vi "Performance Test.vi"() -> ()   [LabVIEW 2021]
uses:
  ChannelCommon/typedef/Benchmark Stats.ctl
  CIFChannels/Typedef/Direction.ctl
  CIF_NIChn_Fifo_U8.lvclass
  D:/dev/Packages/Channel_Manager/src/CIFChannels/CIFChannels.lvclass
  ChannelCommon/typedef/FIFO Config.ctl
  <vilib>/Platform/TimedLoop/XDataNode/timing_clust.ctl
  <vilib>/Platform/TimedLoop/XDataNode/nitl_modes.ctl
  <vilib>/Platform/TimedLoop/XDataNode/wakeup.ctl
  ChannelCommon/typedef/TimeStamps.ctl
  CIFChannels/CIFChannels.lvclass/CIFChannels.ctl
  <vilib>/CIF Foundation/CIF Utilities/Statistics/I64/Stats_I64_CIF_U.lvclass/Stats_I64_CIF_U.ctl
  <vilib>/CIF Foundation/CIF Utilities/DataTypes/Flatten U64.vi
  <vilib>/CIF Foundation/CIF Utilities/Statistics/I64/Get Stats.vi
  <vilib>/Platform/TimedLoop/XDataNode/XDataNode.xnode
  <vilib>/Platform/TimedLoop/XDataNode/XDNodeRunTimeDep.lvlib
  CIFChannels/CIFChannels.lvclass
  ChannelCommon/ChannelCommon.lvlib
panel:
  out "Flatten (us) TO":T1
  out "Channel R/W (us) TO":T1
  out "Flatten (us)":T1
  out "Channel R/W (us)":T1
  out "avg TO":dbl
  out "max TO":dbl
  out "timed out? 3":bool
  out "timed out?":bool
  out "avg channel":dbl
  out "max channel":dbl
  out "pass":bool
  out "error out":errorcluster
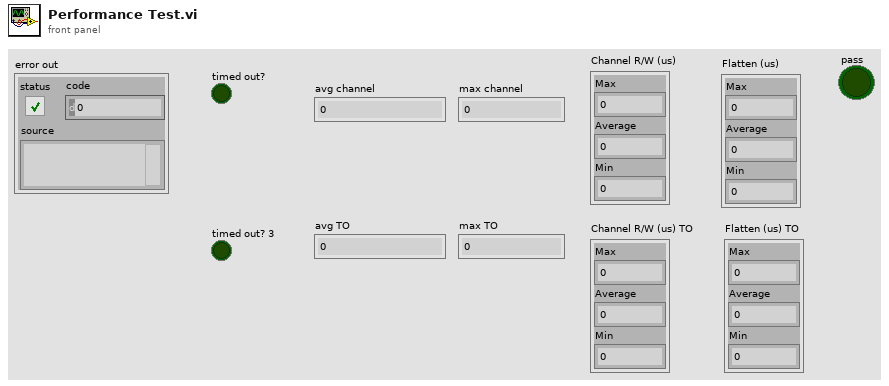
[diagram p1: front panel]
types:
  T1 = typedef "ChannelCommon.lvlib/Benchmark Stats.ctl" = cluster{"Max":i64, "Average":dbl, "Min":i64}
  T2 = typedef "ChannelCommon.lvlib/FIFO Config.ctl" = cluster{"Max Bytes/Msg":u64, "Max Msg/FIFO":u64, "Flags":u64}
  T3 = typedef "CIFChannels.lvclass/Direction.ctl" = enum16{"Publisher", "Subscriber"}
  T4 = typedef "ChannelCommon.lvlib/TimeStamps.ctl" = cluster{"ClockID":u8, "T0":i64, "T_Out":i64}
  T5 = typedef "XDNodeRunTimeDep.lvlib/timing_clust.ctl" = cluster{"Expected End [f-1]":u64, "Actual End [f-1]":u64, "Finished Late? [f-1]":bool, "Expected End [i-1]":u64, "Actual End [i-1]":u64, "Finished Late? [i-1]":bool, "Expected Start [i]":u64, "Actual Start [i]":u64, "Expected Start [f]":u64, "Actual Start [f]":u64, "Source Name":string, "Structure Name":string, "Period":i64, "Deadline":i64, "Offset":i64, "Start":i64, "Priority":i32, "Timeout":i32, "Mode":T6, "Wakeup Reason":T7, "Error":errorcluster, "Source Type":string, "Secondary Source Type":string, "Global End Time":u64, "Global Start Time":u64, "Frame Duration":u64, "Iteration Duration":u64, "Assigned CPU":i32, "I/O Scan Engine Mode":u32}
  T6 = typedef "XDNodeRunTimeDep.lvlib/nitl_modes.ctl" = enum32{"No Change", "Process missed periods, maintain original phase", "Discard missed periods, maintain original phase", "Process missed periods, ignore original phase", "Discard missed periods, ignore original phase"}
  T7 = typedef "XDNodeRunTimeDep.lvlib/wakeup.ctl" = enum32{"Normal", "Aborted", "Asynchronous wakeup", "Timing source error", "Timed loop error", "Timeout"}
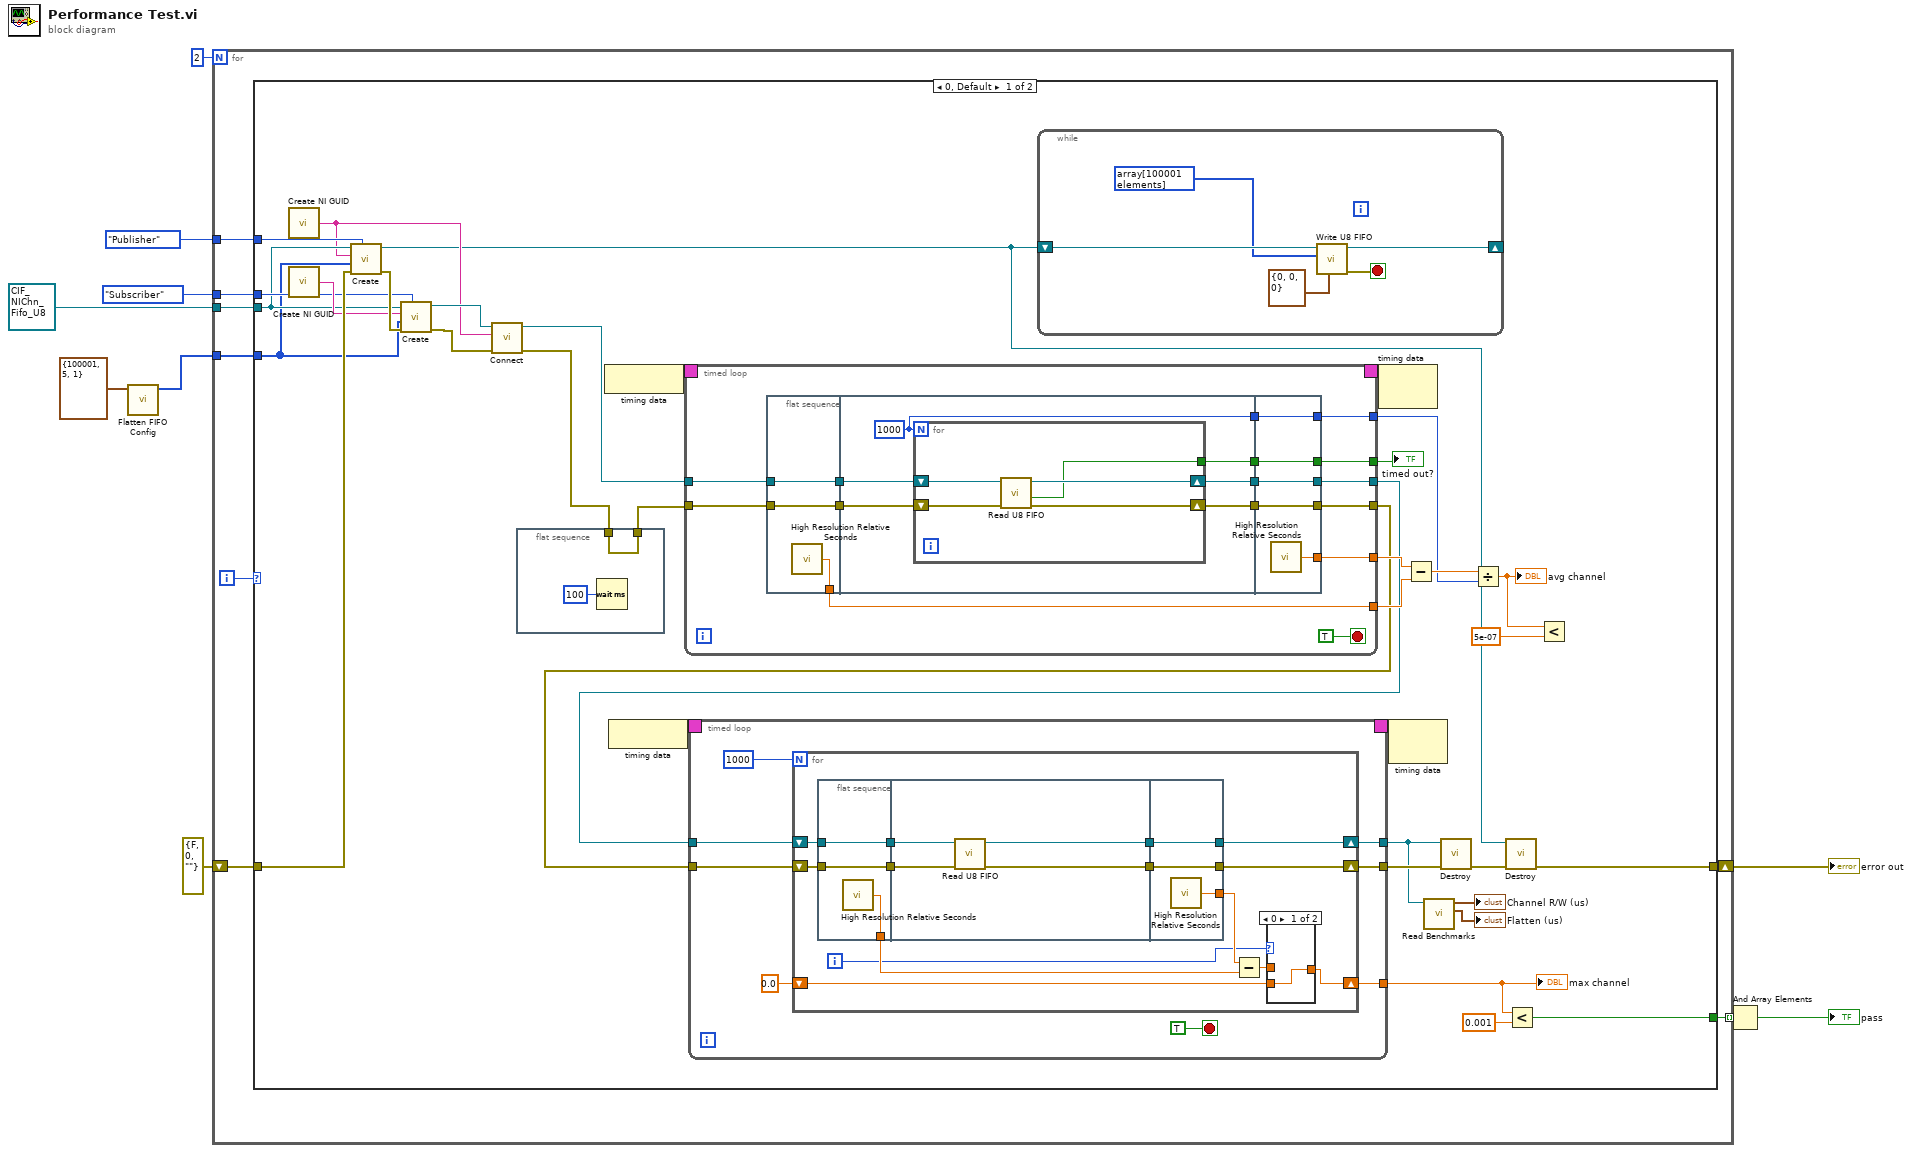
[diagram p0: block diagram]
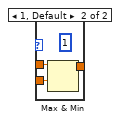
[diagram p2: hidden frame]
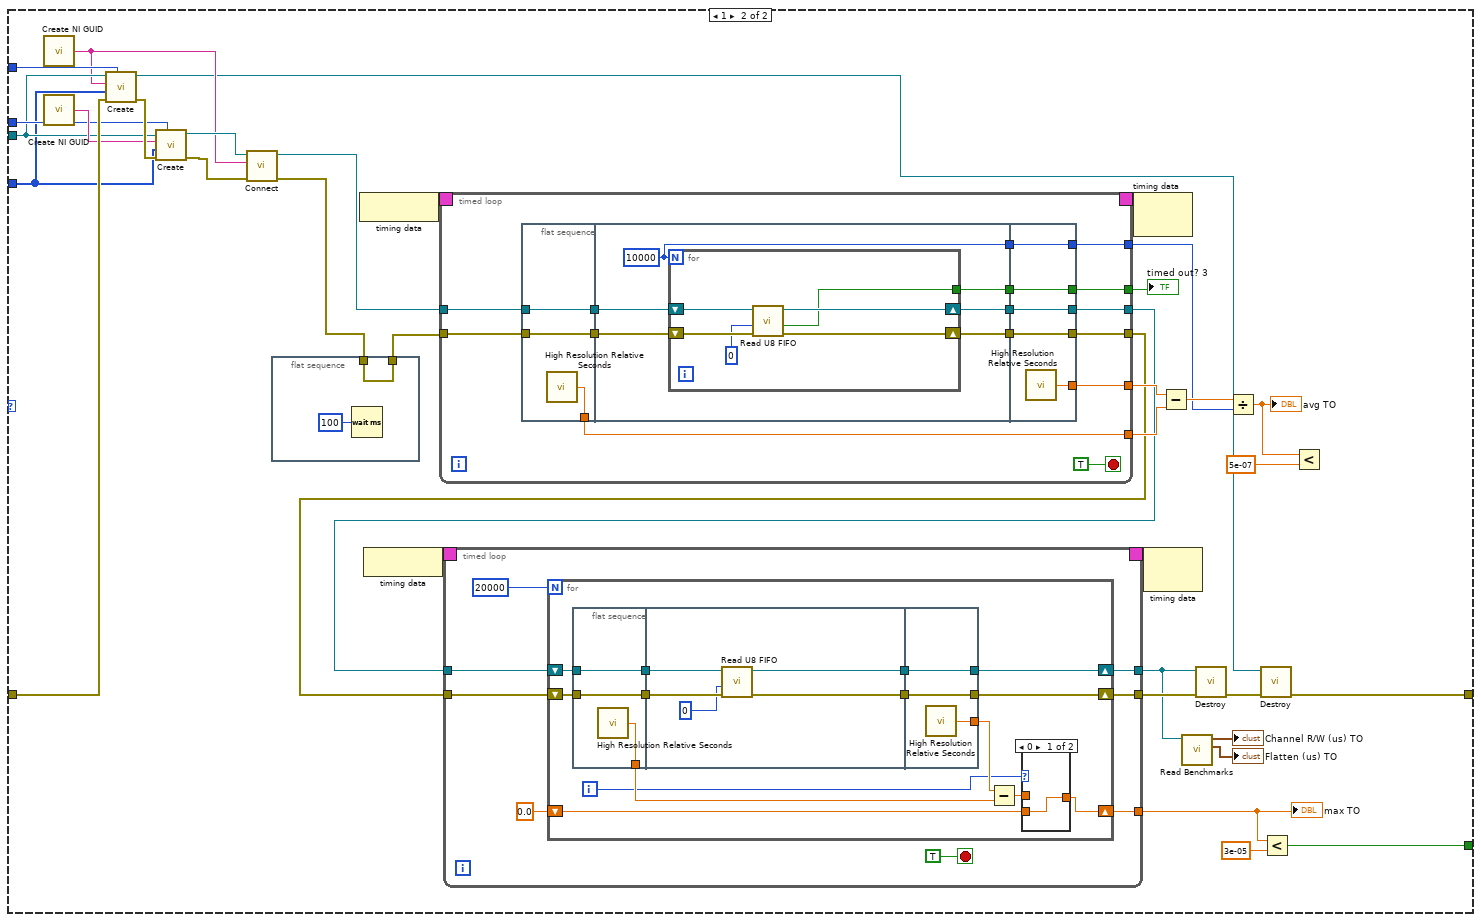
[diagram p3: hidden frame]
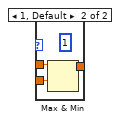
[diagram p4: hidden frame]
diagram:
  n1 = call "Flatten FIFO Config.vi"("FIFO Config in"=T2 {"Max Bytes/Msg"=100001, "Max Msg/FIFO"=5, "Flags"=1}) -> ("Flattened FIFO Config"=w1:u8[])  [unwired: 10 in]
  n2 = for {
    N: 2 -> [_]
    tunnel: [w18] -> w8 mode=indexing
    shift-right: [w17] -> w10
    shift-left: errorcluster {"status"=FALSE, "code"=0, "source"=""} ("error out") -> [w15]
    tunnel: Direction."Publisher" ("Direction") -> [w14]
    tunnel: Direction."Subscriber" ("Direction") -> [w13]
    tunnel: refnum<class "CIF_NIChn_Fifo_U8.lvclass"> refnum ("CIF_NIChn_Fifo_Power.lvclass") -> [w12]
    tunnel: w1 -> [w11]
    i -> [w16]
    n3 = case shown="0, Default" w16 {
      tunnel: [w40 w161] -> w18
      tunnel: [w25 w146] -> w17
      tunnel: w15 -> [w38 w159]
      tunnel: w14 -> [w36 w157]
      tunnel: w13 -> [w35 w156]
      tunnel: w12 -> [w34 w155]
      tunnel: w11 -> [w30 w151]
      frame 0, Default {
        n4 = call <vilib>:"Create NI GUID.vi"() -> ("NI GUID"=w32:string)
        n5 = call <vilib>:"Create NI GUID.vi"() -> ("NI GUID"=w37:string)
        n6 = call-dynamic "Create.vi"("Direction"=w36, "error in (no error)"=w38, "Custom Config Data"=w30, "Name"=w32, "CIFFIFO in"=w34) -> ("error out"=w39:errorcluster, "CIFFIFO out"=w26:refnum<class "CIF_NIChn_Fifo_U8.lvclass">)  [unwired: 5 in]
        n7 = call-dynamic "Create.vi"("Direction"=w35, "error in (no error)"=w39, "Custom Config Data"=w30, "Name"=w37, "CIFFIFO in"=w34) -> ("error out"=w31:errorcluster, "CIFFIFO out"=w33:refnum<class "CIF_NIChn_Fifo_U8.lvclass">)  [unwired: 5 in]
        n8 = call-dynamic "Connect.vi"("error in (no error)"=w31, "Connection Name"=w32, "CIFTag in"=w33) -> ("error out"=w24:errorcluster, "CIFTag out"=w29:refnum<class "CIF_NIChn_Fifo_U8.lvclass">)  [unwired: 7 in]
        n9 = flat-sequence {
          tunnel: w24 -> [w56]
          tunnel: [w56] -> w23
          frame #0 {
            n10 = Wait (ms)(milliseconds to wait=u32 100) -> ()  [unwired: 1 out]
          }
        }
        n11 = node-c288() -> (w54:T5)
        n12 = node-c288() -> (w52:T5)
        n13 = timed-loop {
          timing: w54 -> [_]
          timing-out: [_] -> w53
          tunnel: w29 -> [w116]
          tunnel: w23 -> [w115]
          tunnel: [w111] -> w46
          tunnel: [w109] -> w45
          tunnel: [w107] -> w50
          tunnel: [w106] -> w49
          tunnel: [w105] -> w47
          tunnel: [w103] -> w22
          stop <- TRUE stop-if-true
          n14 = flat-sequence {
            tunnel: w115 -> [w118]
            tunnel: w116 -> [w119]
            tunnel: [w119] -> w113
            tunnel: [w118] -> w112
            tunnel: [w117] -> w106
            tunnel: w113 -> [w125]
            tunnel: w112 -> [w124]
            tunnel: [w123] -> w110
            tunnel: [w122] -> w108
            tunnel: [w121] -> w104
            tunnel: [w120] -> w102
            tunnel: [w135] -> w111
            tunnel: w110 -> [w135]
            tunnel: [w134] -> w109
            tunnel: w108 -> [w134]
            tunnel: [w133] -> w107
            tunnel: [w132] -> w105
            tunnel: w104 -> [w132]
            tunnel: [w131] -> w103
            tunnel: w102 -> [w131]
            frame #0 {
              n15 = call <vilib>:"High Resolution Relative Seconds.vi"() -> ("relative seconds"=w117:dbl)
            }
            frame #1 {
              w121 = 1000
              n16 = for {
                N: w121 -> [_]
                shift-right: [w127] -> w123
                shift-left: w125 -> [w130]
                shift-right: [w128] -> w122
                shift-left: w124 -> [w129]
                tunnel: [w126] -> w120
                n17 = call-dynamic "Read U8 FIFO.vi"("error in (no error)"=w129, "CIFFIFO in"=w130) -> ("error out"=w128:errorcluster, "timed out?"=w126:bool, "CIFFIFO out"=w127:refnum<class "CIF_NIChn_Fifo_U8.lvclass">)  [unwired: 5 in, 2 out]
              }
            }
            frame #2 {
              n18 = call <vilib>:"High Resolution Relative Seconds.vi"() -> ("relative seconds"=w133:dbl)
            }
          }
        }
        "timed out?" <- w22
        n19 = timed-loop {
          timing: w52 -> [_]
          timing-out: [_] -> w51
          tunnel: w46 -> [w69]
          tunnel: w45 -> [w68]
          tunnel: [w66] -> w21
          tunnel: [w65] -> w28
          tunnel: [w62] -> w42
          stop <- TRUE stop-if-true
          n20 = for {
            N: 1000 -> [_]
            shift-right: [w78] -> w66
            shift-left: w69 -> [w80]
            shift-right: [w77] -> w65
            shift-left: w68 -> [w79]
            shift-right: [w72] -> w62
            shift-left: 0.0 -> [w73]
            i -> [w71]
            n21 = flat-sequence {
              tunnel: w79 -> [w89]
              tunnel: w80 -> [w90]
              tunnel: [w90] -> w83
              tunnel: [w89] -> w82
              tunnel: [w88] -> w75
              tunnel: w83 -> [w94]
              tunnel: w82 -> [w93]
              tunnel: [w91] -> w81
              tunnel: [w92] -> w70
              tunnel: [w97] -> w78
              tunnel: w81 -> [w97]
              tunnel: [w96] -> w77
              tunnel: [w95] -> w76
              tunnel: w70 -> [w96]
              frame #0 {
                n22 = call <vilib>:"High Resolution Relative Seconds.vi"() -> ("relative seconds"=w88:dbl)
              }
              frame #1 {
                n23 = call-dynamic "Read U8 FIFO.vi"("error in (no error)"=w93, "CIFFIFO in"=w94) -> ("error out"=w92:errorcluster, "CIFFIFO out"=w91:refnum<class "CIF_NIChn_Fifo_U8.lvclass">)  [unwired: 5 in, 3 out]
              }
              frame #2 {
                n24 = call <vilib>:"High Resolution Relative Seconds.vi"() -> ("relative seconds"=w95:dbl)
              }
            }
            n25 = Subtract(x=w76, y=w75) -> (x-y=w74:dbl)
            n26 = case shown="0" w71 {
              tunnel: w74 -> [_ w87]
              tunnel: w73 -> [w84 w86]
              tunnel: [w84 w85] -> w72
              frame 0 {
              }
              frame 1, Default {
                (unwired) u32 1 ("milliseconds to wait")
                n27 = Max & Min(x=w87, y=w86) -> (max(x,y)=w85:dbl)  [unwired: 1 out]
              }
            }
          }
        }
        "max channel" <- w42
        n28 = while {
          shift-right: [w58] -> _
          shift-left: w26 -> [w61]
          stop <- w59 stop-if-true
          n29 = call-dynamic "Write U8 FIFO.vi"("FIFO Timestamps"=T4 {"ClockID"=0, "T0"=0, "T_Out"=0}, "Data in"=u8[] array[100001 elements] ("U8 Data"), "CIFFIFO in"=w61) -> ("error out"=w59:errorcluster, "CIFFIFO out"=w58:refnum<class "CIF_NIChn_Fifo_U8.lvclass">)  [unwired: 5 in, 2 out]
        }
        n30 = node-c288(w53) -> ()  [unwired: 1 out]
        n31 = node-c288(w51) -> ()  [unwired: 1 out]
        n32 = Subtract(x=w50, y=w49) -> (x-y=w48:dbl)
        n33 = call "Read Benchmarks.vi"("CIFChannels in"=w21) -> ("Flatten (us)"=→"Flatten (us)":T1, "Channel R/W (us)"=→"Channel R/W (us)":T1)  [unwired: 9 in]
        n34 = call-dynamic "Destroy.vi"("error in (no error)"=w28, "CIFFIFO in"=w21) -> ("error out"=w27:errorcluster)  [unwired: 8 in, 1 out]
        n35 = Divide(x=w48, y=w47) -> (x/y=w44:dbl)
        "avg channel" <- w44
        n36 = call-dynamic "Destroy.vi"("error in (no error)"=w27, "CIFFIFO in"=w26) -> ("error out"=w25:errorcluster)  [unwired: 8 in, 1 out]
        n37 = Less?(x=w42, y=0.001) -> (x < y?=w40:bool)
        n38 = Less?(x=w44, y=5e-07) -> ()  [unwired: 1 out]
      }
      frame 1 {
        n39 = call <vilib>:"Create NI GUID.vi"() -> ("NI GUID"=w153:string)
        n40 = call <vilib>:"Create NI GUID.vi"() -> ("NI GUID"=w158:string)
        n41 = call-dynamic "Create.vi"("Direction"=w157, "error in (no error)"=w159, "Custom Config Data"=w151, "Name"=w153, "CIFFIFO in"=w155) -> ("error out"=w160:errorcluster, "CIFFIFO out"=w147:refnum<class "CIF_NIChn_Fifo_U8.lvclass">)  [unwired: 5 in]
        n42 = call-dynamic "Create.vi"("Direction"=w156, "error in (no error)"=w160, "Custom Config Data"=w151, "Name"=w158, "CIFFIFO in"=w155) -> ("error out"=w152:errorcluster, "CIFFIFO out"=w154:refnum<class "CIF_NIChn_Fifo_U8.lvclass">)  [unwired: 5 in]
        n43 = call-dynamic "Connect.vi"("error in (no error)"=w152, "Connection Name"=w153, "CIFTag in"=w154) -> ("error out"=w145:errorcluster, "CIFTag out"=w150:refnum<class "CIF_NIChn_Fifo_U8.lvclass">)  [unwired: 7 in]
        n44 = flat-sequence {
          tunnel: w145 -> [w177]
          tunnel: [w177] -> w144
          frame #0 {
            n45 = Wait (ms)(milliseconds to wait=u32 100) -> ()  [unwired: 1 out]
          }
        }
        n46 = node-c288() -> (w175:T5)
        n47 = node-c288() -> (w173:T5)
        n48 = timed-loop {
          timing: w175 -> [_]
          timing-out: [_] -> w174
          tunnel: w150 -> [w233]
          tunnel: w144 -> [w232]
          tunnel: [w228] -> w167
          tunnel: [w226] -> w166
          tunnel: [w224] -> w171
          tunnel: [w223] -> w170
          tunnel: [w222] -> w168
          tunnel: [w220] -> w143
          stop <- TRUE stop-if-true
          n49 = flat-sequence {
            tunnel: w232 -> [w235]
            tunnel: w233 -> [w236]
            tunnel: [w236] -> w230
            tunnel: [w235] -> w229
            tunnel: [w234] -> w223
            tunnel: w230 -> [w242]
            tunnel: w229 -> [w241]
            tunnel: [w240] -> w227
            tunnel: [w239] -> w225
            tunnel: [w238] -> w221
            tunnel: [w237] -> w219
            tunnel: [w253] -> w228
            tunnel: w227 -> [w253]
            tunnel: [w252] -> w226
            tunnel: w225 -> [w252]
            tunnel: [w251] -> w224
            tunnel: [w250] -> w222
            tunnel: w221 -> [w250]
            tunnel: [w249] -> w220
            tunnel: w219 -> [w249]
            frame #0 {
              n50 = call <vilib>:"High Resolution Relative Seconds.vi"() -> ("relative seconds"=w234:dbl)
            }
            frame #1 {
              w238 = 10000
              n51 = for {
                N: w238 -> [_]
                shift-right: [w245] -> w240
                shift-left: w242 -> [w248]
                shift-right: [w246] -> w239
                shift-left: w241 -> [w247]
                tunnel: [w244] -> w237
                n52 = call-dynamic "Read U8 FIFO.vi"("error in (no error)"=w247, "Timeout (ms)"=0, "CIFFIFO in"=w248) -> ("error out"=w246:errorcluster, "timed out?"=w244:bool, "CIFFIFO out"=w245:refnum<class "CIF_NIChn_Fifo_U8.lvclass">)  [unwired: 4 in, 2 out]
              }
            }
            frame #2 {
              n53 = call <vilib>:"High Resolution Relative Seconds.vi"() -> ("relative seconds"=w251:dbl)
            }
          }
        }
        "timed out? 3" <- w143
        n54 = timed-loop {
          timing: w173 -> [_]
          timing-out: [_] -> w172
          tunnel: w167 -> [w185]
          tunnel: w166 -> [w184]
          tunnel: [w182] -> w140
          tunnel: [w181] -> w149
          tunnel: [w178] -> w163
          stop <- TRUE stop-if-true
          n55 = for {
            N: 20000 -> [_]
            shift-right: [w194] -> w182
            shift-left: w185 -> [w196]
            shift-right: [w193] -> w181
            shift-left: w184 -> [w195]
            shift-right: [w188] -> w178
            shift-left: 0.0 -> [w189]
            i -> [w187]
            n56 = flat-sequence {
              tunnel: w195 -> [w205]
              tunnel: w196 -> [w206]
              tunnel: [w206] -> w199
              tunnel: [w205] -> w198
              tunnel: [w204] -> w191
              tunnel: w199 -> [w211]
              tunnel: w198 -> [w209]
              tunnel: [w210] -> w197
              tunnel: [w208] -> w186
              tunnel: [w214] -> w194
              tunnel: w197 -> [w214]
              tunnel: [w213] -> w193
              tunnel: [w212] -> w192
              tunnel: w186 -> [w213]
              frame #0 {
                n57 = call <vilib>:"High Resolution Relative Seconds.vi"() -> ("relative seconds"=w204:dbl)
              }
              frame #1 {
                n58 = call-dynamic "Read U8 FIFO.vi"("error in (no error)"=w209, "Timeout (ms)"=0, "CIFFIFO in"=w211) -> ("error out"=w208:errorcluster, "CIFFIFO out"=w210:refnum<class "CIF_NIChn_Fifo_U8.lvclass">)  [unwired: 4 in, 3 out]
              }
              frame #2 {
                n59 = call <vilib>:"High Resolution Relative Seconds.vi"() -> ("relative seconds"=w212:dbl)
              }
            }
            n60 = Subtract(x=w192, y=w191) -> (x-y=w190:dbl)
            n61 = case shown="0" w187 {
              tunnel: w190 -> [_ w203]
              tunnel: w189 -> [w200 w202]
              tunnel: [w200 w201] -> w188
              frame 0 {
              }
              frame 1, Default {
                (unwired) u32 1 ("milliseconds to wait")
                n62 = Max & Min(x=w203, y=w202) -> (max(x,y)=w201:dbl)  [unwired: 1 out]
              }
            }
          }
        }
        "max TO" <- w163
        n63 = node-c288(w174) -> ()  [unwired: 1 out]
        n64 = node-c288(w172) -> ()  [unwired: 1 out]
        n65 = Subtract(x=w171, y=w170) -> (x-y=w169:dbl)
        n66 = call "Read Benchmarks.vi"("CIFChannels in"=w140) -> ("Flatten (us)"=→"Flatten (us) TO":T1, "Channel R/W (us)"=→"Channel R/W (us) TO":T1)  [unwired: 9 in]
        n67 = call-dynamic "Destroy.vi"("error in (no error)"=w149, "CIFFIFO in"=w140) -> ("error out"=w148:errorcluster)  [unwired: 8 in, 1 out]
        n68 = Divide(x=w169, y=w168) -> (x/y=w165:dbl)
        "avg TO" <- w165
        n69 = call-dynamic "Destroy.vi"("error in (no error)"=w148, "CIFFIFO in"=w147) -> ("error out"=w146:errorcluster)  [unwired: 8 in, 1 out]
        n70 = Less?(x=w163, y=3e-05) -> (x < y?=w161:bool)
        n71 = Less?(x=w165, y=5e-07) -> ()  [unwired: 1 out]
      }
    }
  }
  "error out" <- w10
  n72 = And Array Elements(Boolean array=w8) -> (logical AND=→"pass":bool)
